vi "Read Attributes.vi"(11 "SentTimerToParent Msg":refnum<class "SentTimerToParent Msg.lvclass">) -> (2 "Payload":T1)   [LabVIEW 2020, in "SentTimerToParent Msg.lvclass"]
uses:
  SentTimerToParent Msg.lvclass
  SentTimerToParent Msg.lvclass/SentTimerToParent Msg.ctl
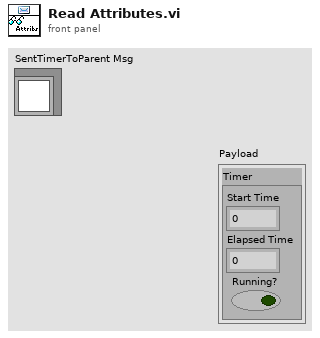
[diagram p1: front panel]
types:
  T1 = cluster{"Timer":cluster{"Start Time":i32, "Elapsed Time":i32, "Running?":bool}}
  T2 = cluster{"Start Time":i32, "Elapsed Time":i32, "Running?":bool}
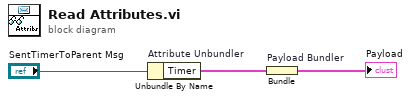
[diagram p0: block diagram]
diagram:
  n1 = Unbundle By Name "Attribute Unbundler"("SentTimerToParent Msg") -> ("Timer"=w1:T2)
  n2 = Bundle "Payload Bundler"("Timer"=w1) -> (→"Payload":T1)  [unwired: 1 in]
